vi "Path to String.vi"(3 "Path":path) -> (1 "Path String":string)   [LabVIEW 2020, in "CDM-Config.lvlib"]
uses:
  CDM-Config.lvlib
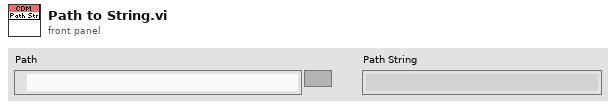
[diagram p1: front panel]
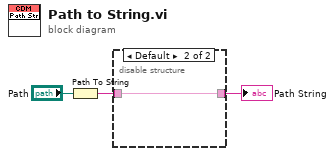
[diagram p0: block diagram]
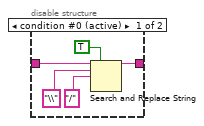
[diagram p2: hidden frame]
diagram:
  n1 = Path To String(path="Path") -> (string=w2:string)
  n2 = disable-structure shown="Default" {
    disable-tunnel: w2 -> [w8 w9]
    disable-tunnel: [w4 w9] -> w1
    frame condition #0 (active) {
      n3 = Search and Replace String(replace all?=TRUE ("replace all? (F)"), input string=w8, search string="\\", replace string="/" ("search string")) -> (result string=w4:string)  [unwired: 4 in, 3 out]
    }
    frame condition #1 {
    }
  }
  "Path String" <- w1
